vi "XYZStage-Read speed setting command (ver 2).vi"(8 "error in (no error)":errorcluster, 10 "XYZ Stage data to queue":T1={"Command"=enum."Initialize", "Channel"="Z", "X"=0.0, "Y"=0.0, "Z"=0.0, "Speed"=0, "Zero"=FALSE, "Use acknowledgement?"=TRUE} {"Speed" format="Speed= %.0f"; "Z" format="Z= %#_g"; "Y" format="Y= %#_g"; "X" format="X= %#_g"}, 11 "XYZ Stage Control.lvclass":refnum<class "XYZ Stage Control.lvclass">) -> (0 "error out":errorcluster, 3 "XYZ Stage Control.lvclass":refnum<class "XYZ Stage Control.lvclass">)   [LabVIEW 2020]
doc: "Reads the XYZ Stage coordinates"
uses:
  Typedefs/XYZ stage data.ctl
  Typedefs/XYZ stage states.ctl
  Typedefs/XYZ channel ring.ctl
  XYZ Stage Control/XYZ Stage Control.lvclass
  Typedefs/Command acknowledgment states.ctl
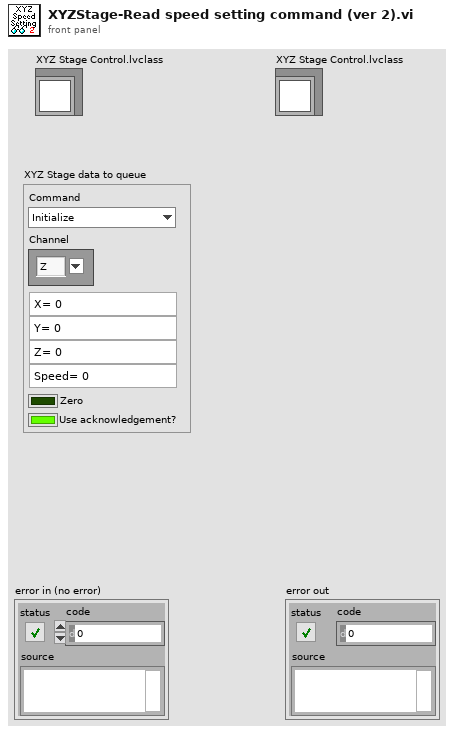
[diagram p1: front panel]
types:
  T1 = typedef "XYZ stage data.ctl" = cluster{"Command":T2, "Channel":T3, "X":sgl, "Y":sgl, "Z":sgl, "Speed":i32, "Zero":bool, "Use acknowledgement?":bool}
  T2 = typedef "XYZ stage states.ctl" = enum16{"Dequeue", "Initialize", "Read Position", "Read Speed Setting", "Move", "Set Max Speed", "Reset Axis", "Stop all movement"}
  T3 = typedef "XYZ channel ring.ctl" = string
  T4 = typedef "Command acknowledgment states.ctl" = enum16{"Acknowledge", "Wait for acknowledgment", "Release queue"}
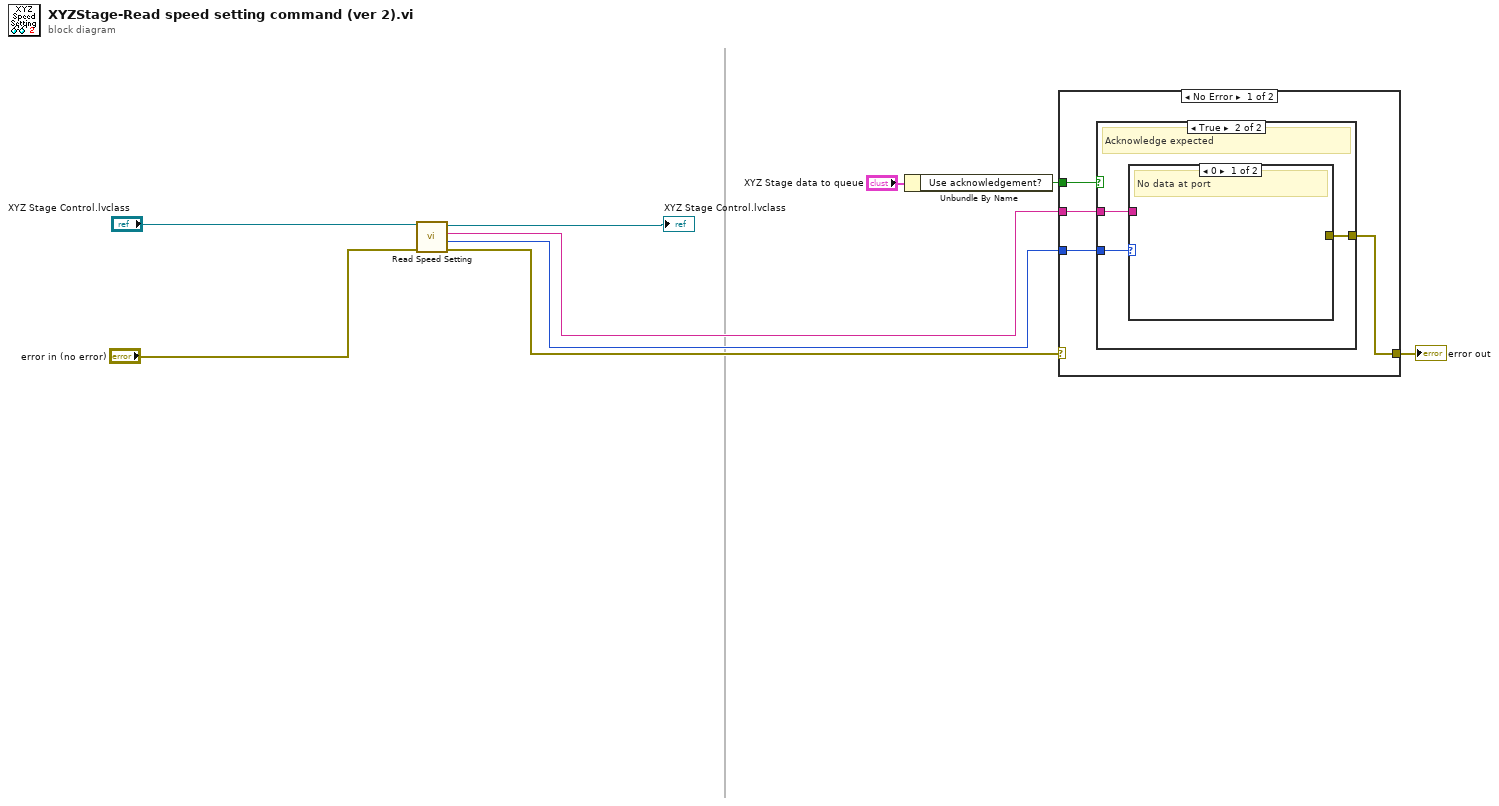
[diagram p0: block diagram]
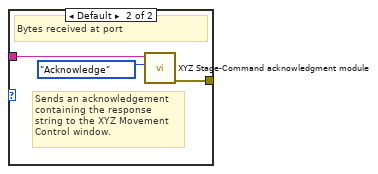
[diagram p3: hidden frame]
diagram:
  n1 = call-dynamic "Read Speed Setting.vi"("error in (no error)"="error in (no error)", "XYZ Stage Control in"="XYZ Stage Control.lvclass") -> ("error out"=w5:errorcluster, "bytes read"=w3:u32, "Speed Setting"=w6:string, "XYZ Stage Control out"=→"XYZ Stage Control.lvclass":refnum<class "XYZ Stage Control.lvclass">)  [unwired: 6 in]
  n2 = Unbundle By Name("XYZ Stage data to queue") -> ("Use acknowledgement?"=w8:bool)
  n3 = case shown="No Error" w5 {
    selector: w5 -> [_ w20]
    tunnel: w8 -> [w13 _]
    tunnel: w6 -> [w12 _]
    tunnel: [w11 w20] -> w4
    tunnel: w3 -> [w10 _]
    frame No Error {
      n4 = case shown="True" w13 {
        tunnel: w12 -> [_ w16]
        tunnel: [_ w15] -> w11
        tunnel: w10 -> [_ w14]
        frame False {
          # "No acknowledgement expected"
        }
        frame True {
          # "Acknowledge expected"
          n5 = case shown="0" w14 {
            tunnel: w16 -> [_ w18]
            tunnel: [_ w17] -> w15
            frame 0 {
              # "No data at port"
            }
            frame Default {
              # "Sends an acknowledgement containing the response string to the XYZ Movement Control window."
              # "Bytes received at port"
              n6 = call "XYZ Stage-Command acknowledgment module.vi"("State"=Command_acknowledgment_states."Acknowledge", "Acknowledgement Message in"=w18) -> ("error out"=w17:errorcluster)  [unwired: 7 in, 2 out]
            }
          }
        }
      }
    }
    frame Error {
    }
  }
  "error out" <- w4
